vi "Read val.vi"(8 "error in (no error)":errorcluster, 11 "PowerSupply MSG in":refnum<class "PowerSupply MSG.lvclass">) -> (0 "error out":errorcluster, 2 "val":u8, 3 "PowerSupply MSG out":refnum<class "PowerSupply MSG.lvclass">)   [LabVIEW 2014, in "Controller.lvlib" / "PowerSupply MSG.lvclass"]
uses:
  PowerSupply MSG.lvclass
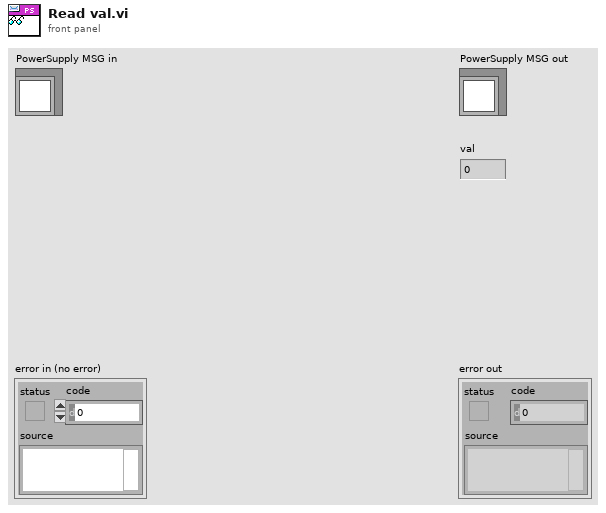
[diagram p1: front panel]
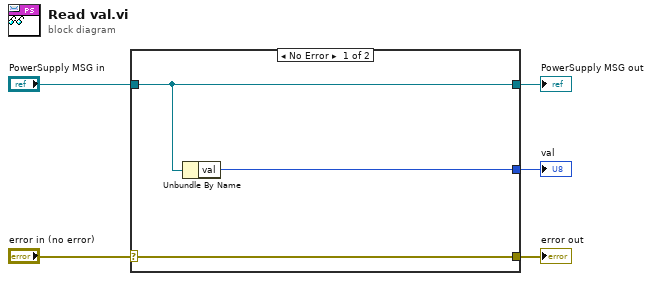
[diagram p0: block diagram]
diagram:
  n1 = case shown="No Error" "error in (no error)" {
    selector: "error in (no error)" -> [w8 w9]
    tunnel: [w8 w9] -> w4
    tunnel: [w7 w10] -> w2
    tunnel: "PowerSupply MSG in" -> [w7 w10]
    tunnel: [w6 _] -> w1
    frame No Error {
      n2 = Unbundle By Name(w7) -> ("val"=w6:u8)
    }
    frame Error {
    }
  }
  "error out" <- w4
  "PowerSupply MSG out" <- w2
  "val" <- w1
